vi "Write acquisition configuration.vi"(8 "error in (no error)":errorcluster, 11 "Channel in":refnum<class "Channel.lvclass">) -> (0 "error out":errorcluster, 3 "Channel out":refnum<class "Channel.lvclass">)   [LabVIEW 2018, in "Channel.lvclass"]
uses:
  Channel.lvclass
  Channel.lvclass/Channel.ctl
  Simulated_CCD_Camera/Simulated Camera.lvclass
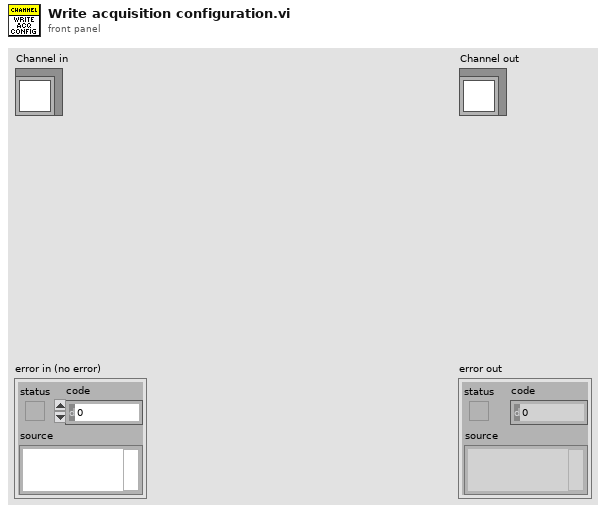
[diagram p1: front panel]
types:
  T1 = cluster{"EXPTIME":errorcluster, "#FRAMES":errorcluster, "#CYCLES":errorcluster, "WAVEPLATE_POS":errorcluster, "TEMP":errorcluster, "COOLER_POWER_STATUS":errorcluster, "SUFFIX":errorcluster}
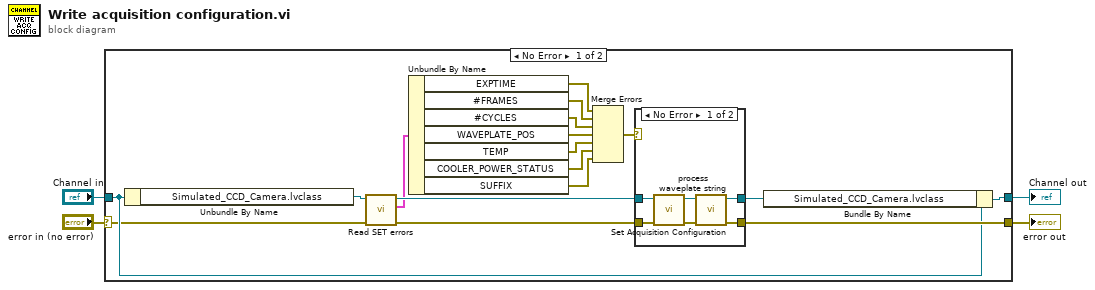
[diagram p0: block diagram]
diagram:
  n1 = case shown="No Error" "error in (no error)" {
    selector: "error in (no error)" -> [w5 w31]
    tunnel: [w20 w31] -> w3
    tunnel: [w19 w30] -> w1
    tunnel: "Channel in" -> [w6 w30]
    frame No Error {
      n2 = Unbundle By Name(w6) -> ("Simulated_CCD_Camera.lvclass"=w18:refnum<class "Simulated Camera.lvclass">)
      n3 = call-dynamic "Read SET errors.vi"("error in (no error)"=w5, "Simulated Camera in"=w18) -> ("error out"=w16:errorcluster, "SET errors"=w15:T1, "Simulated Camera out"=w17:refnum<class "Simulated Camera.lvclass">)  [unwired: 7 in]
      n4 = Unbundle By Name(w15) -> ("EXPTIME"=w14:errorcluster, "#FRAMES"=w13:errorcluster, "#CYCLES"=w12:errorcluster, "WAVEPLATE_POS"=w11:errorcluster, "TEMP"=w10:errorcluster, "COOLER_POWER_STATUS"=w9:errorcluster, "SUFFIX"=w8:errorcluster)
      n5 = Merge Errors(w14, w13, w12, w11, w10, w9, w8) -> (w7:errorcluster)
      n6 = case shown="No Error" w7 {
        tunnel: w17 -> [w26 w29]
        tunnel: w16 -> [w27 w28]
        tunnel: [w25 w28] -> w20
        tunnel: [w24 w29] -> w21
        frame No Error {
          n7 = call-dynamic "Set Acquisition Configuration.vi"("error in (no error)"=w27, "CCDCamera in"=w26) -> ("error out"=w22:errorcluster, "CCDCamera out"=w23:refnum<class "Simulated Camera.lvclass">)  [unwired: 8 in]
          n8 = call "process waveplate string.vi"("error in (no error)"=w22, "Simulated_CCD_Camera in"=w23) -> ("error out"=w25:errorcluster, "Simulated_CCD_Camera out"=w24:refnum<class "Simulated Camera.lvclass">)  [unwired: 8 in]
        }
        frame Error {
        }
      }
      n9 = Bundle By Name(cluster=w6, "Simulated_CCD_Camera.lvclass"=w21) -> (w19:refnum<class "Channel.lvclass">)
    }
    frame Error {
    }
  }
  "error out" <- w3
  "Channel out" <- w1
